vi "GetCurrentImage.vi"(2 "Image":T1, 4 "tracker":u64) -> (0 "copy of current CUDA image":T1(plugin-control), 1 "tracker":u64)   [LabVIEW 2011]
uses:
  <vilib>/vision/Image Controls.llb/IMAQ Image.ctl
  cudatrack-debug.dll
panel:
  out "targetImage":u64
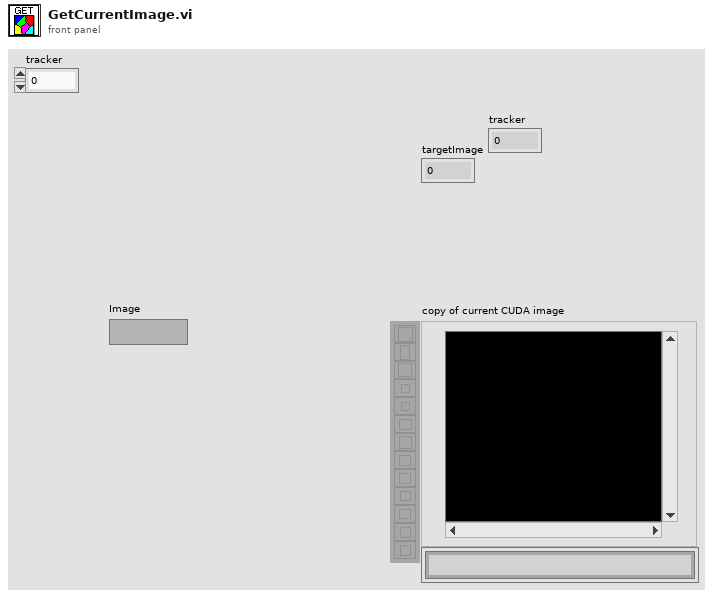
[diagram p1: front panel]
types:
  T1 = typedef "IMAQ Image.ctl" = refnum<image>
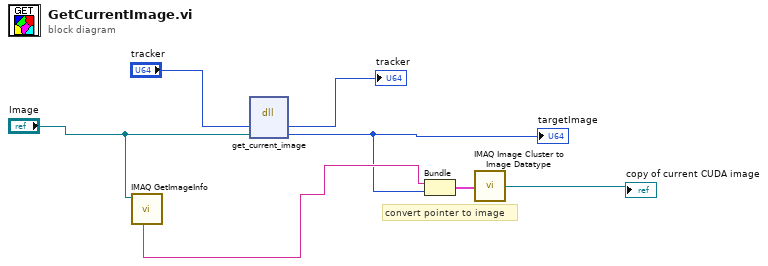
[diagram p0: block diagram]
diagram:
  # "convert pointer to image"
  n1 = call "IMAQ GetImageInfo"("Image"="Image") -> ("Image Name"=w4:string)  [unwired: 3 in, 7 out]
  n2 = dll-call lib="D:/jcnossen1/cudaqi-tracker/cudatrack/cudatrack-debug.dll" fn="get_current_image"("trackerInstance"="tracker", "targetImage"="Image") -> ("trackerInstance"=→"tracker":u64, "targetImage"=w3:u64)  [unwired: 4 in, 2 out]
  "targetImage" <- w3
  n3 = Bundle("Image Name"=w4, "targetImage"=w3) -> (w6:cluster{"Image Name":string, "targetImage":u64})  [unwired: 1 in]
  n4 = call <vilib>:"IMAQ Image Cluster to Image Datatype.vi"("Image"=w6) -> ("Image (dup)"=→"copy of current CUDA image":T1)
